vi "Actor Core.vi"(8 "error in":errorcluster, 11 "DigitiserActor in":refnum<class "DigitiserActor.lvclass">) -> (0 "error out":errorcluster, 3 "Actor out":refnum<class "Actor.lvclass">)   [LabVIEW 2019, in "DigitiserActor.lvlib" / "DigitiserActor.lvclass"]
doc: "(<B>Filename</B>: Actor Framework.lvlib:Actor.lvclass:Actor Core.vi)\n\nReceives messages to the actor, reacts to them, and initiates any error handling that may shut the actor down.\n\nDescendant classes may override this VI to append parallel tasks for the actor to complete while it handles messages. Overrides use the Call Parent Method node."
uses:
  DigitiserActor.lvclass
  C:/Program Files (x86)/National Instruments/LabVIEW 2019/vi.lib/ActorFramework/Actor/Actor.lvclass
  <vilib>/ActorFramework/Actor/Actor.lvclass
  <vilib>/ActorFramework/Actor/Actor.lvclass/Actor.ctl
  <vilib>/ActorFramework/Message Enqueuer/Message Enqueuer.lvclass/Message Enqueuer.ctl
  <vilib>/ActorFramework/Message Enqueuer/Init from Existing Queue.vi
  <vilib>/ActorFramework/Message Enqueuer/Enqueue.vi
  <vilib>/ActorFramework/Stop Msg/Stop Msg.lvclass
  C:/Program Files (x86)/National Instruments/LabVIEW 2019/vi.lib/ActorFramework/Message/Message.lvclass
  <vilib>/ActorFramework/Message Priority Queue/Priority Enqueue.vi
  <vilib>/ActorFramework/Message Enqueuer/Message Enqueuer.lvclass
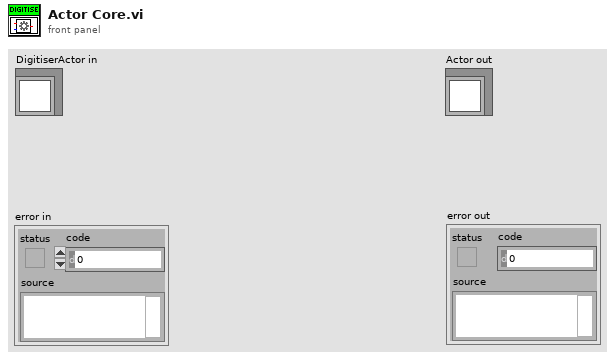
[diagram p1: front panel]
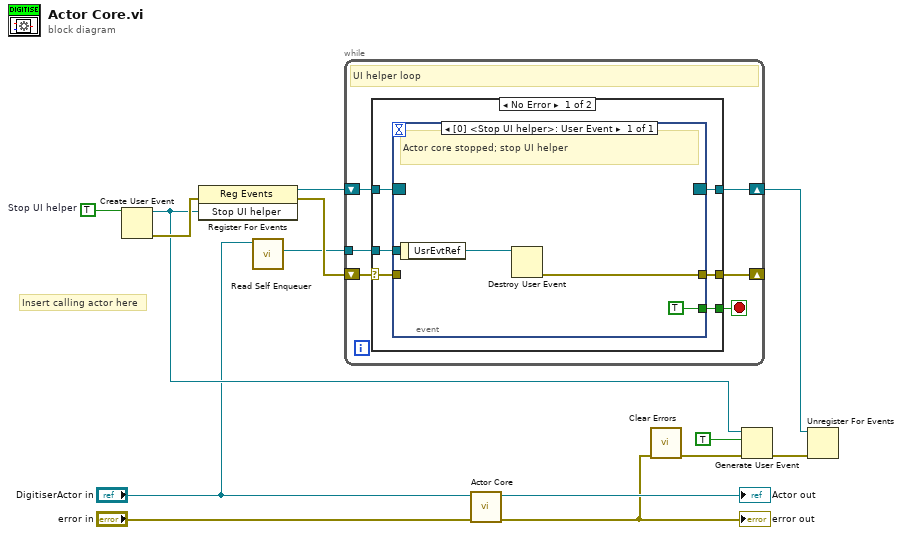
[diagram p0: block diagram]
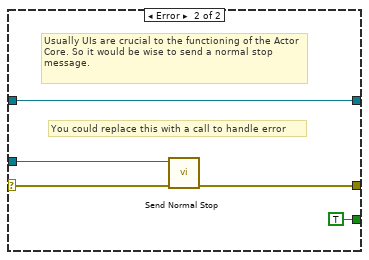
[diagram p2: hidden frame]
diagram:
  w11 = TRUE  # Stop UI helper
  # "Insert calling actor here"
  n1 = Create User Event(user event datatype=w11) -> (user event=w7:refnum<user-event>, error out=w10:errorcluster)  [unwired: 1 in]
  n2 = register-events(error in=w10, w7) -> (reference out=w12:refnum<event-registration>, error out=w4:errorcluster)  [unwired: 1 in]
  n3 = call <vilib>:"Read Self Enqueuer.vi"("Actor"="DigitiserActor in") -> ("Self Enqueuer"=w3:refnum<class "Message Enqueuer.lvclass">)  [unwired: 10 in]
  n4 = while {
    shift-right: [w19] -> w9
    shift-left: w12 -> [w20]
    shift-right: [w16] -> _
    shift-left: w4 -> [w17]
    tunnel: w3 -> [w15]
    stop <- w18 stop-if-true
    # "UI helper loop"
    n5 = case shown="No Error" w17 {
      selector: w17 -> [w23 w32]
      tunnel: w20 -> [w26 w34]
      tunnel: [w25 w34] -> w19
      tunnel: [w24 TRUE] -> w18
      tunnel: [w22 w31] -> w16
      tunnel: w15 -> [w21 w30]
      frame No Error {
        n6 = event shown="[0] <Stop UI helper>: User Event" {
          selector: w26 -> [_]
          dyn-events: [_] -> w25
          timeout: _ -> [_]
          tunnel: [TRUE] -> w24
          tunnel: w23 -> [_]
          tunnel: [w27] -> w22
          tunnel: w21 -> [_]
          event User Event {
            # "Actor core stopped; stop UI helper"
            n7 = event-data() -> ("UsrEvtRef"=w28:refnum<user-event>)  [unwired: 1 in]
            n8 = Destroy User Event(user event=w28) -> (error out=w27:errorcluster)  [unwired: 1 in]
          }
        }
      }
      frame Error {
        # "You could replace this with a call to handle error"
        # "Usually UIs are crucial to the functioning of the Actor Core. So it would be wise to send a normal stop message."
        n9 = call <vilib>:"Send Normal Stop.vi"("error in (no error)"=w32, "Message Enqueuer"=w30) -> ("error out"=w31:errorcluster)  [unwired: 9 in]
      }
    }
  }
  n10 = call-parent "Actor Core.vi"("error in"="error in", "Actor in"="DigitiserActor in") -> ("error out"=w2:errorcluster, "Actor out"=→"Actor out":refnum<class "Actor.lvclass">)  [unwired: 8 in]
  "error out" <- w2
  n11 = call <vilib>:"Clear Errors.vi"("error in (no error)"=w2) -> ("error out"=w5:errorcluster)  [unwired: 5 in, 1 out]
  n12 = Generate User Event(user event=w7, event data cluster=TRUE ("event data"), error in=w5) -> (error out=w8:errorcluster)  [unwired: 1 in, 1 out]
  n13 = Unregister For Events(event registration refnum=w9, error in=w8) -> ()  [unwired: 1 out]
